vi "DBLToSGL.vi"(5 "Number":dbl) -> (1 "Single precision float":sgl, 2 "Overflow?":bool, 3 "Exact conversion?":bool)   [LabVIEW 2017, in "GPOverflow.lvlib"]
doc: "Converts <B>Number</B> to SGL keeping track of numeric overflow and exactness of conversion.\n\n<B>Exact conversion?</B> will be True only if a conversion back into the original data type of <B>Number</B> will yield the exact same number, i.e. no precision was lost during the conversion.\n\n<B>Overflow?</B> will be True if positive or negative overflow occurred. The numeric output will saturate in case of overflow.\n\nThis VI is inlined.\n\nSteen Schmidt\nGPower\n6/3 2013"
uses:
  GPOverflow.lvlib
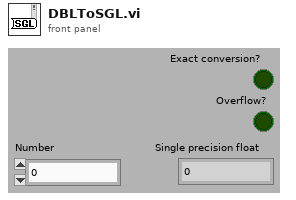
[diagram p1: front panel]
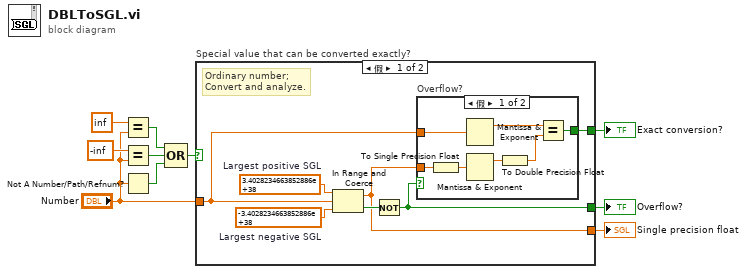
[diagram p0: block diagram]
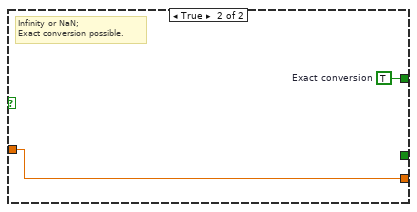
[diagram p3: hidden frame]
diagram:
  n1 = Equal?(x=inf ("Number"), y="Number") -> (x = y?=w4:bool)
  n2 = Equal?(x=-inf ("Number"), y="Number") -> (x = y?=w5:bool)
  n3 = Not A Number/Path/Refnum?(number/path/refnum="Number") -> (NaN/Path/Refnum?=w1:bool)
  n4 = Compound Arithmetic op=OR(w4, w5, w1) -> (w3:bool)
  n5 = case "Special value that can be converted exactly?" shown="假" w3 {
    tunnel: [w14 _] -> w10
    tunnel: [w11 w25] -> w9
    tunnel: "Number" -> [w13 w25]
    tunnel: [w12 w26] -> w8
    frame False {
      w15 = -3.4028234663852886e+38  # Largest negative SGL
      w16 = 3.4028234663852886e+38  # Largest positive SGL
      # "Ordinary number;\nConvert and analyze."
      n6 = In Range and Coerce(upper limit=w16, x=w13, lower limit=w15) -> (coerced(x)=w11:dbl, In Range?=w17:bool)
      n7 = Not(x=w17) -> (.not. x?=w14:bool)
      n8 = case "Overflow?" shown="假" w14 {
        tunnel: w11 -> [w19 _]
        tunnel: w13 -> [w24 _]
        tunnel: [w20 _] -> w12
        frame False {
          n9 = To Single Precision Float(number=w19) -> (single precision float=w18:sgl)
          n10 = Mantissa & Exponent(0:w24) -> (1:w21:dbl)  [unwired: 1 out]
          n11 = Mantissa & Exponent(0:w18) -> (1:w23:sgl)  [unwired: 1 out]
          n12 = To Double Precision Float(number=w23) -> (double precision float=w22:dbl)
          n13 = Equal?(x=w21, y=w22) -> (x = y?=w20:bool)
        }
        frame True {
        }
      }
    }
    frame True {
      w26 = TRUE  # Exact conversion
      # "Infinity or NaN;\nExact conversion possible."
    }
  }
  "Single precision float" <- w9
  "Overflow?" <- w10
  "Exact conversion?" <- w8
